vi "Initialise_File.vi"(9 "<File Name>.txt (Don't add extension)":string, 10 "Data Save Path:":path=path "C:/Users/labpc/Documents/ProbeStation Users Data") -> (0 "error out":errorcluster, 2 "Actual Save Path":path, 3 "refnum out":refnum<file>)   [LabVIEW 2021]
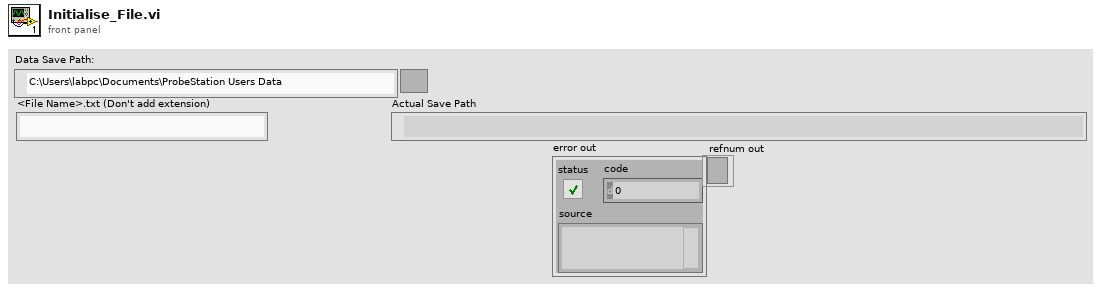
[diagram p1: front panel]
types:
  T1 = enum16{"open", "replace", "create", "open or create", "replace or create", "replace or create with confirmation"}
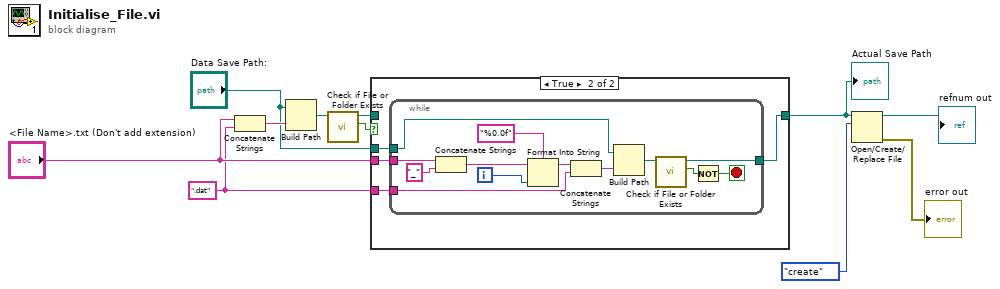
[diagram p0: block diagram]
diagram:
  w5 = ".dat"
  n1 = Concatenate Strings("<File Name>.txt (Don't add extension)", w5) -> (w11:string)
  n2 = Build Path(base path="Data Save Path:", name or relative path=w11) -> (appended path=w10:path)
  n3 = call <vilib>:"Check if File or Folder Exists.vi"("path"=w10) -> ("file or folder exists?"=w9:bool, "dup path"=w8:path)  [unwired: 8 in, 1 out]
  n4 = case shown="True" w9 {
    tunnel: [w12 w13] -> w3
    tunnel: w8 -> [w12 _]
    tunnel: "Data Save Path:" -> [_ w14]
    tunnel: "<File Name>.txt (Don't add extension)" -> [_ w16]
    tunnel: w5 -> [_ w15]
    frame False {
    }
    frame True {
      n5 = while {
        tunnel: w16 -> [w19]
        tunnel: w15 -> [w24]
        tunnel: w14 -> [w22]
        tunnel: [w20] -> w13
        i -> [w26]
        stop <- w28 stop-if-true
        n6 = Concatenate Strings(w19, "_" ("string")) -> (w18:string)
        n7 = Format Into String(format string="%0.0f", initial string=w18, w26) -> (resulting string=w25:string)  [unwired: 1 in, 1 out]
        n8 = Concatenate Strings(w25, w24) -> (w23:string)
        n9 = Build Path(base path=w22, name or relative path=w23) -> (appended path=w21:path)
        n10 = call <vilib>:"Check if File or Folder Exists.vi"("path"=w21) -> ("file or folder exists?"=w29:bool, "dup path"=w20:path)  [unwired: 8 in, 1 out]
        n11 = Not(x=w29) -> (.not. x?=w28:bool)
      }
    }
  }
  "Actual Save Path" <- w3
  n12 = Open/Create/Replace File(file path (use dialog)=w3, operation (0:open)=T1."create") -> (refnum out=→"refnum out":refnum<file>, error out=→"error out":errorcluster)  [unwired: 4 in, 1 out]
